vi "test6.vi"   [LabVIEW 2012]
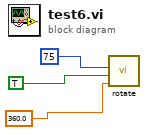
[diagram p0: block diagram]
diagram:
  n1 = call "rotate.vi"("degrees to  rotate"=360.0, "right(T)/left(F)"=TRUE, "power"=u16 75) -> ()  [unwired: 8 in, 1 out]
